vi "RTS Add Setup Info.vi"(8 "Error In":errorcluster, 10 "Setup Info Array":string[][](array[string])=[["FILENAME:", ""], ["TR NUMBER:", ""], ["LAB ID:", ""], ["TEST TYPE:", ""], ["MODEL NUMBER:", ""], ["SERIAL NUMBER:", ""], ["STATION ID:", ""], ["ENGINEER:", ""], ["TECHNICIAN:", ""], ["WATER PRESSURE (PSI):", ""], ["AMBINENT RH (%):", ""], ["SUPPLY VOLTAGE (V)", ""], ["FREQUENCY (HZ)", ""], ["BUILD:", ""], ["LABVIEW SOFTWARE VERSION:", ""], ["COMPUTER NAME:", ""], ["COMPUTER IP ADDRESS:", ""], ["COMMENTS", ""], ["LOAD RUN NUMBER", "0"], ["AMBIENT TEMPERATURE (F):", ""]], 11 "file path":path) -> (0 "Error Out":errorcluster)   [LabVIEW 2016]
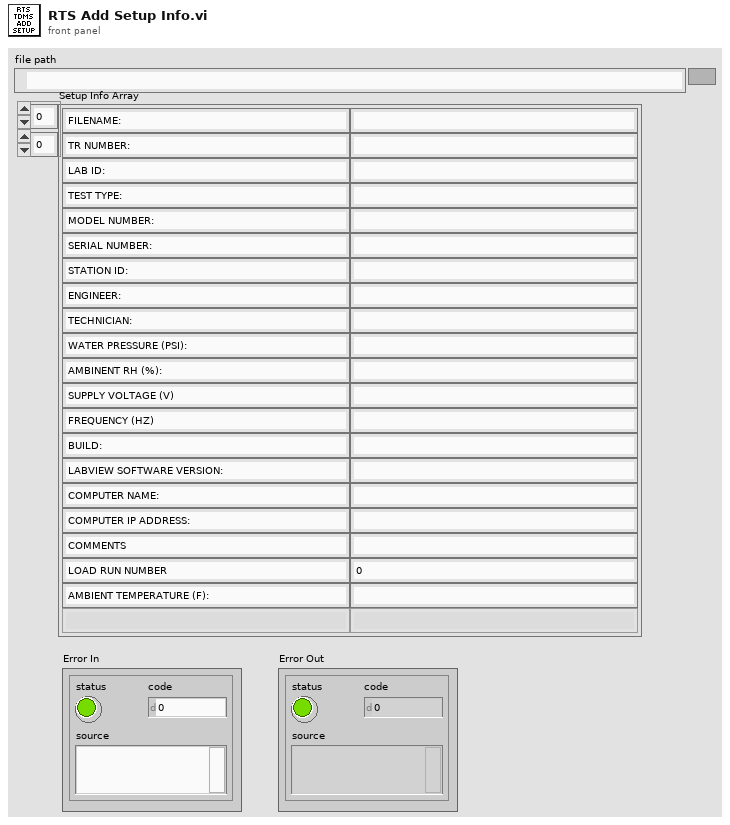
[diagram p1: front panel]
types:
  T1 = enum16{"open", "open or create", "create or replace", "create", "open (read-only)"}
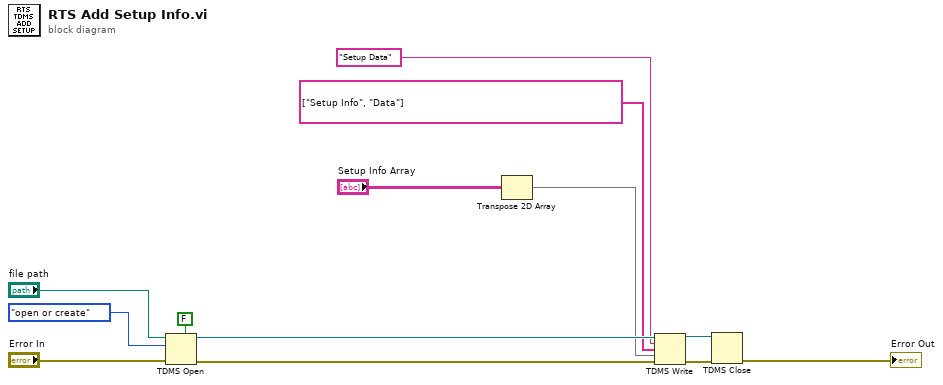
[diagram p0: block diagram]
diagram:
  n1 = TDMS Open(5:FALSE ("create index file? (T)"), 8:"Error In", 10:T1."open or create" ("operation (0:open)"), 11:"file path") -> (0:w13:errorcluster, 3:w10:refnum<k34>)  [unwired: 3 in]
  n2 = Transpose 2D Array(2D array="Setup Info Array") -> (transposed array=w4:string[][])
  n3 = TDMS Write(0:w10, 5:"Setup Data" ("group name in (Untitled)"), 7:string[] ["Setup Info", "Data"] ("channel name(s) in (Untitled)"), 9:w4, 11:w13) -> (4:w11:refnum<k34>, 15:w12:errorcluster)  [unwired: 1 in, 2 out]
  n4 = TDMS Close(8:w12, 11:w11) -> (0:→"Error Out":errorcluster)  [unwired: 1 out]
